vi "Set Port Map.vi"(8 "error in":errorcluster, 10 "port map":u32, 11 "port ref":T1 format="%.0x") -> (0 "error out":errorcluster, 3 "port ref out":T1 format="%.0x")   [LabVIEW 2020, in "AIM ARINC 664 Scripting.lvlib"]
uses:
  AIM ARINC 664 Scripting.lvlib
  <vilib>/NI VeriStand/Custom Device API/Custom Device API.lvlib
  <vilib>/NI VeriStand/Custom Device API/Set Item Property (U32).vi
  Constants.vi
  <vilib>/NI VeriStand/Custom Device API/Custom Device Item Ref.ctl
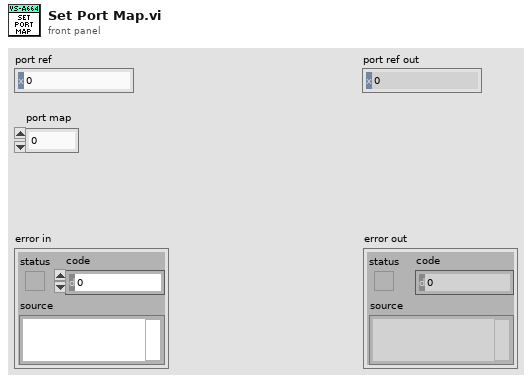
[diagram p1: front panel]
types:
  T1 = typedef "Custom Device API.lvlib/Custom Device Item Ref.ctl" = u64
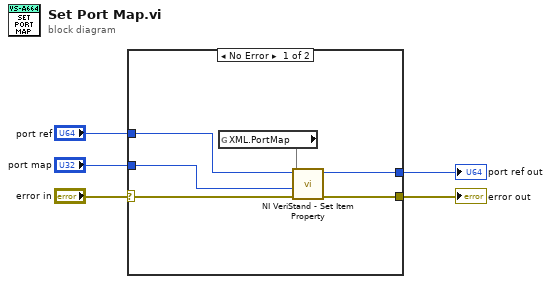
[diagram p0: block diagram]
diagram:
  n1 = case shown="No Error" "error in" {
    selector: "error in" -> [w6 w13]
    tunnel: "port ref" -> [w10 w12]
    tunnel: [w9 w13] -> w4
    tunnel: "port map" -> [w8 _]
    tunnel: [w7 w12] -> w2
    frame No Error {
      n2 = global read "Constants.vi" "XML.PortMap"() -> (w11)
      n3 = call-poly <vilib>:"NI VeriStand - Set Item Property.vi"("error in (no error)"=w6, "Value"=w8, "Property Name"=w11, "Item Ref in"=w10) -> ("error out"=w9:errorcluster, "Item Ref out"=w7:T1)  [unwired: 5 in, 1 out]
    }
    frame Error {
    }
  }
  "error out" <- w4
  "port ref out" <- w2
